vi "Build_Array.vi"() -> ()   [LabVIEW 2024]
panel:
  out "appended array":dbl[](array[numeric])
  in  "Numeric 4":dbl
  in  "Numeric 3":dbl
  in  "Numeric 2":dbl
  in  "Numeric":dbl
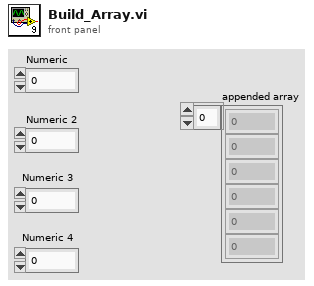
[diagram p1: front panel]
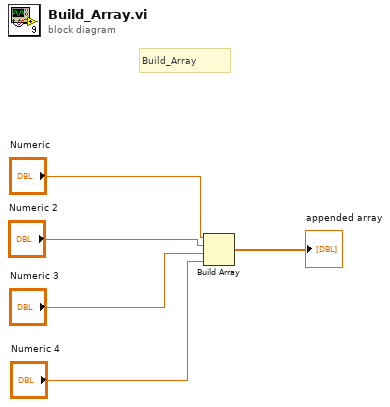
[diagram p0: block diagram]
diagram:
  # "Build_Array"
  n1 = Build Array("Numeric", "Numeric 2", "Numeric 3", "Numeric 4") -> (→"appended array":dbl[])
